vi "ReadSF.vi"(0 "ID_sensor0\nBlue":u16, 2 "connection IDs":T1, 5 "ID_sensor0\nRed":u16, 7 "ID_sensor1\nBlue":u16, 9 "ID_sensor1\nRed":u16) -> (4 "Line sensors\nBlue":dbl[](array[numeric]), 6 "Wheel turns\nBlue":dbl, 8 "Line sensors\nRed":dbl[](array[numeric]), 10 "Wheel turns\nRed":dbl, 13 "Distances\nBlue":dbl[](array[numeric]), 14 "Distances\nRed":dbl[](array[numeric]))   [LabVIEW 2010]
panel:
  out "message":string
  out "payload":string
  out "header":string
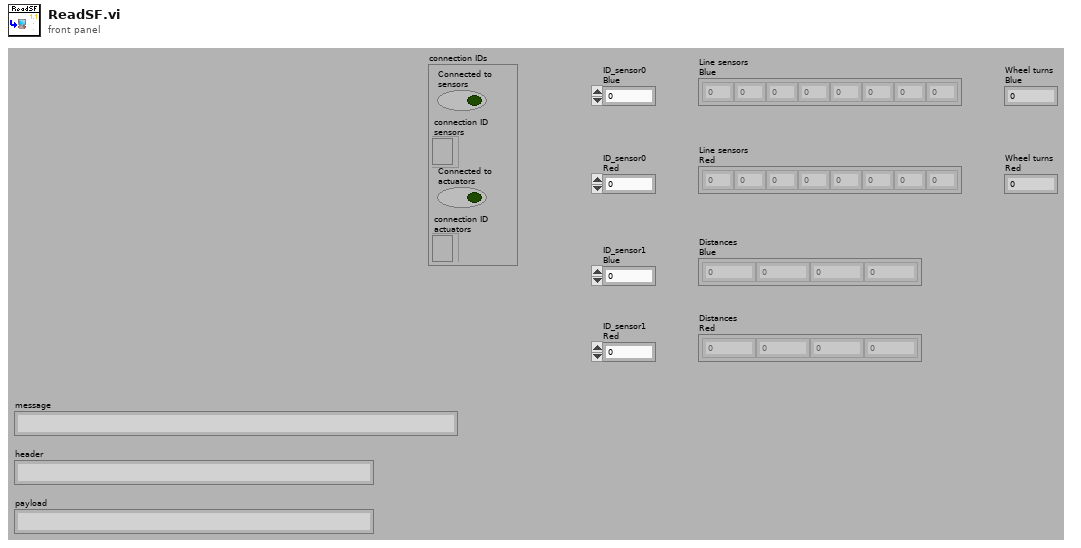
[diagram p1: front panel]
types:
  T1 = cluster{"Connected to\nsensors":bool, "connection ID\nsensors":refnum<k5>, "Connected to\nactuators":bool, "connection ID\nactuators":refnum<k5>}
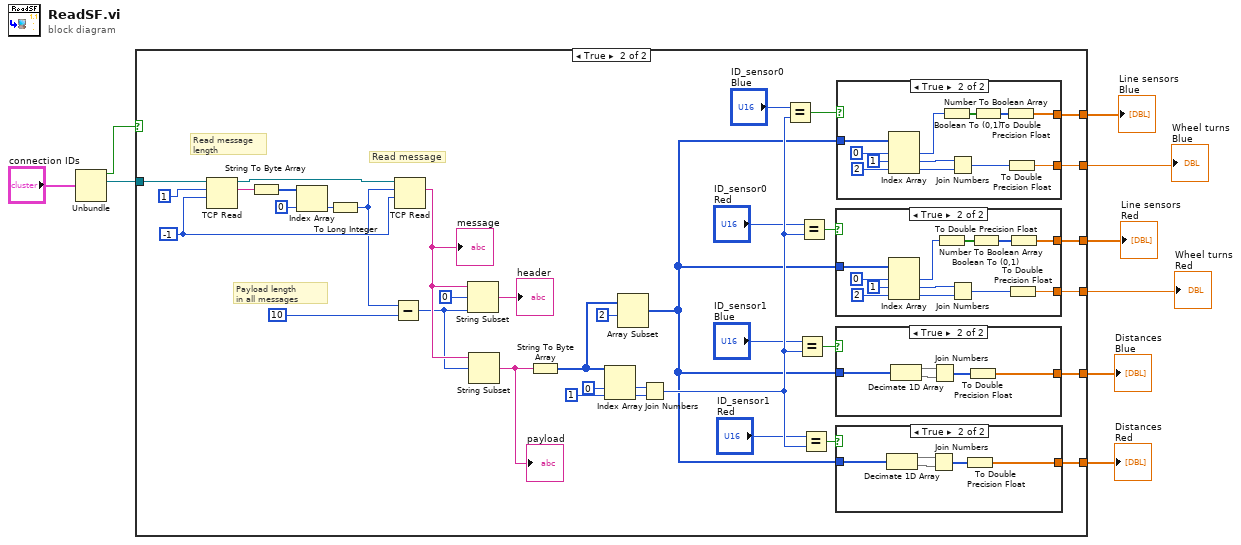
[diagram p0: block diagram]
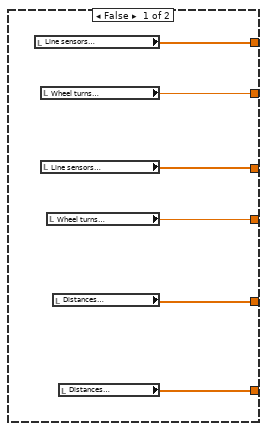
[diagram p2: hidden frame]
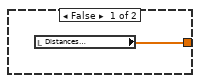
[diagram p3: hidden frame]
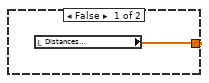
[diagram p4: hidden frame]
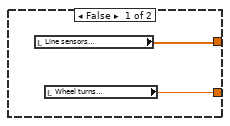
[diagram p5: hidden frame]
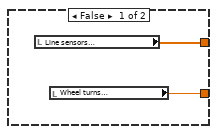
[diagram p6: hidden frame]
diagram:
  n1 = Unbundle("connection IDs") -> ("Connected to\nsensors"=w8:bool, "connection ID\nsensors"=w7:refnum<k5>)  [unwired: 2 out]
  n2 = case shown="True" w8 {
    tunnel: w7 -> [_ w36]
    tunnel: [w15 w22] -> w4
    tunnel: [w14 w21] -> w6
    tunnel: [w13 w20] -> w3
    tunnel: [w12 w19] -> w5
    tunnel: [w11 w18] -> w2
    tunnel: [w10 w16] -> w1
    frame False {
      n3 = local read "Line sensors\nBlue"() -> (w15:dbl[])
      n4 = local read "Wheel turns\nBlue"() -> (w14:dbl)
      n5 = local read "Line sensors\nRed"() -> (w13:dbl[])
      n6 = local read "Wheel turns\nRed"() -> (w12:dbl)
      n7 = local read "Distances\nBlue"() -> (w11:dbl[])
      n8 = local read "Distances\nRed"() -> (w10:dbl[])
    }
    frame True {
      w47 = -1 ("timeout ms (25000)")
      # "Payload length\nin all messages"
      # "Read message"
      # "Read message\nlength"
      n9 = TCP Read(connection ID=w36, bytes to read=1, 9:w47) -> (connection ID out=w48:refnum<k5>, data out=w45:string)  [unwired: 2 in, 1 out]
      n10 = String To Byte Array(string=w45) -> (unsigned byte array=w44:u8[])
      n11 = Index Array(array=w44, index=0) -> (element=w42:u8)
      n12 = To Long Integer(number=w42) -> (32bit integer=w40:i32)
      n13 = Subtract(x=w40, y=10) -> (x-y=w38:i32)
      n14 = TCP Read(connection ID=w48, bytes to read=w40, 9:w47) -> (data out=w39:string)  [unwired: 2 in, 2 out]
      "message" <- w39
      n15 = String Subset(string=w39, offset (0)=0, length (rest)=w38) -> (substring=→"header":string)
      n16 = String Subset(string=w39, offset (0)=w38) -> (substring=w49:string)  [unwired: 1 in]
      "payload" <- w49
      n17 = String To Byte Array(string=w49) -> (unsigned byte array=w24:u8[])
      n18 = Index Array(array=w24, index #1=0, index #2=1) -> (element #1=w35:u8, element #2=w34:u8)
      n19 = Array Subset(array=w24, index=2) -> (w17:u8[])  [unwired: 1 in]
      n20 = Join Numbers(hi=w35, lo=w34) -> ((hi.lo)=w28:u16)
      n21 = Equal?(x="ID_sensor0\nBlue", y=w28) -> (x = y?=w33:bool)
      n22 = Equal?(x="ID_sensor1\nBlue", y=w28) -> (x = y?=w30:bool)
      n23 = Equal?(x="ID_sensor0\nRed", y=w28) -> (x = y?=w31:bool)
      n24 = Equal?(x="ID_sensor1\nRed", y=w28) -> (x = y?=w29:bool)
      n25 = case shown="True" w31 {
        tunnel: w17 -> [_ w72]
        tunnel: [w66 w69] -> w20
        tunnel: [w65 w67] -> w19
        frame False {
          n26 = local read "Line sensors\nRed"() -> (w66:dbl[])
          n27 = local read "Wheel turns\nRed"() -> (w65:dbl)
        }
        frame True {
          n28 = Index Array(array=w72, index #1=0 ("index"), index #2=1 ("index"), index #3=2 ("index")) -> (element #1=w76:u8, element #2=w77:u8, element #3=w78:u8)
          n29 = Number To Boolean Array(number=w76) -> (Boolean array=w71:bool[])
          n30 = Join Numbers(hi=w77, lo=w78) -> ((hi.lo)=w68:u16)
          n31 = Boolean To (0,1)(Boolean=w71) -> (0, 1=w70:i16[])
          n32 = To Double Precision Float(number=w68) -> (double precision float=w67:dbl)
          n33 = To Double Precision Float(number=w70) -> (double precision float=w69:dbl[])
        }
      }
      n34 = case shown="True" w30 {
        tunnel: w17 -> [_ w64]
        tunnel: [w59 w60] -> w18
        frame False {
          n35 = local read "Distances\nBlue"() -> (w59:dbl[])
        }
        frame True {
          n36 = Decimate 1D Array(w64) -> (w63:u8[], w62:u8[])
          n37 = Join Numbers(hi=w63, lo=w62) -> ((hi.lo)=w61:u16[])
          n38 = To Double Precision Float(number=w61) -> (double precision float=w60:dbl[])
        }
      }
      n39 = case shown="True" w29 {
        tunnel: w17 -> [_ w56]
        tunnel: [w53 w54] -> w16
        frame False {
          n40 = local read "Distances\nRed"() -> (w53:dbl[])
        }
        frame True {
          n41 = Decimate 1D Array(w56) -> (w58:u8[], w57:u8[])
          n42 = Join Numbers(hi=w58, lo=w57) -> ((hi.lo)=w55:u16[])
          n43 = To Double Precision Float(number=w55) -> (double precision float=w54:dbl[])
        }
      }
      n44 = case shown="True" w33 {
        tunnel: w17 -> [_ w92]
        tunnel: [w80 w83] -> w22
        tunnel: [w79 w81] -> w21
        frame False {
          n45 = local read "Line sensors\nBlue"() -> (w80:dbl[])
          n46 = local read "Wheel turns\nBlue"() -> (w79:dbl)
        }
        frame True {
          n47 = Index Array(array=w92, index #1=0 ("index"), index #2=1 ("index"), index #3=2 ("index")) -> (element #1=w88:u8, element #2=w87:u8, element #3=w86:u8)
          n48 = Number To Boolean Array(number=w88) -> (Boolean array=w85:bool[])
          n49 = Join Numbers(hi=w87, lo=w86) -> ((hi.lo)=w82:u16)
          n50 = Boolean To (0,1)(Boolean=w85) -> (0, 1=w84:i16[])
          n51 = To Double Precision Float(number=w84) -> (double precision float=w83:dbl[])
          n52 = To Double Precision Float(number=w82) -> (double precision float=w81:dbl)
        }
      }
    }
  }
  "Wheel turns\nBlue" <- w6
  "Wheel turns\nRed" <- w5
  "Line sensors\nBlue" <- w4
  "Line sensors\nRed" <- w3
  "Distances\nBlue" <- w2
  "Distances\nRed" <- w1
